vi "SavedSettingsSetIcon.vi"(8 "error in (no error)":errorcluster, 9 "Restore SubItems":bool=TRUE, 10 "Tag":string, 11 "TreeControl in":refnum<vi>) -> (0 "error out":errorcluster, 3 "reference out":refnum<vi>)   [LabVIEW 2020]
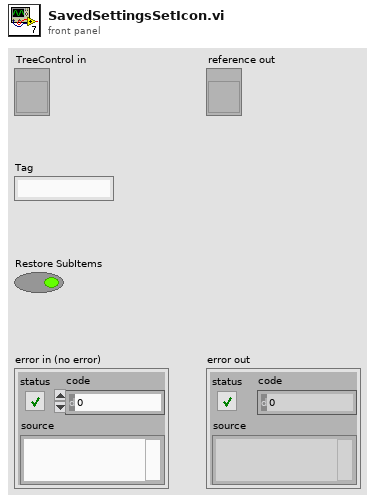
[diagram p1: front panel]
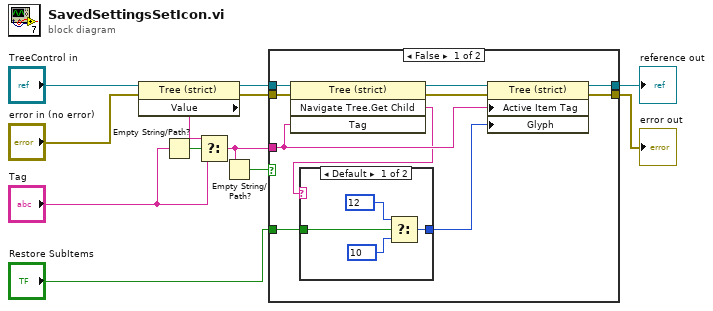
[diagram p0: block diagram]
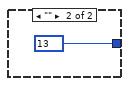
[diagram p2: hidden frame]
diagram:
  n1 = property class="Tree (strict)"(reference="TreeControl in", error in="error in (no error)") -> (reference out=w11:refnum<vi>, error out=w10:errorcluster, "Value"=w6:string)
  n2 = Empty String/Path?(string/path="Tag") -> (empty?=w4:bool)
  n3 = Select(t=w6, s=w4, f="Tag") -> (s? t:f=w3:string)
  n4 = Empty String/Path?(string/path=w3) -> (empty?=w2:bool)
  n5 = case shown="False" w2 {
    tunnel: w11 -> [w20 w29]
    tunnel: w10 -> [w17 w28]
    tunnel: [w21 w28] -> w9
    tunnel: [w22 w29] -> w8
    tunnel: w3 -> [w16 _]
    tunnel: "Restore SubItems" -> [w14 _]
    frame False {
      n6 = invoke class="Tree (strict)" method="Navigate Tree.Get Child"(reference=w20, error in=w17, "Tag"=w16) -> (reference out=w19:refnum<vi>, error out=w18:errorcluster, "Navigate Tree:Get Child"=w15:string)  [unwired: 1 in, 1 out]
      n7 = case shown="Default" w15 {
        tunnel: w14 -> [w24 _]
        tunnel: [w23 13] -> w13
        frame Default {
          n8 = Select(t=12, s=w24, f=10) -> (s? t:f=w23:i32)
        }
        frame "" {
        }
      }
      n9 = property class="Tree (strict)"(reference=w19, error in=w18, "Active Item Tag"=w16, "Glyph"=w13) -> (reference out=w22:refnum<vi>, error out=w21:errorcluster)
    }
    frame True {
    }
  }
  "error out" <- w9
  "reference out" <- w8
